vi "Autonomous Independent.vi"   [LabVIEW 2017]
doc: "This VI is called when autonomous begins, and will automatically be terminated when autonomous ends. You can carry out timed or sensor driven robot movement independently without needing to return to the caller."
uses:
  <vilib>/Rock Robotics/WPI/Utilities/WPI_GetSetVariantRefNum.vi
  <vilib>/Rock Robotics/Network Tables/NT Read String.vi
  Robot Global Data.vi
  <vilib>/Rock Robotics/Network Tables/NT Write Numeric Array.vi
  <vilib>/Rock Robotics/WPI/RobotDrive/WPI_RobotDriveMecanumDrive_Cartesian.vi
panel:
  # "Be sure to right-click and choose Data Operations>>Make Current Value default if you want to save the array values with the VI"
types:
  T1 = typedef "WPI_JoystickDevRef.ctl" = cluster{"Device":T2}
  T2 = typedef "WPI_JoystickDeviceEnum.ctl" = enum16{"USB 0", "USB 1", "USB 2", "USB 3", "USB 4", "USB 5"}
  T3 = typedef "WPI_RobotDriveDevRef.ctl" = cluster{"DevStatus":errorcluster, "Motors[]":T4[], "Square Inputs":bool, "Max Output":dbl}
  T4 = typedef "WPI_MotorControlDeviceRef.ctl" = cluster{"DeviceStatus":errorcluster, "Type":T5, "PWM":cluster{"PWM Channel":T6, "DeadBand":T7}, "CAN":cluster{"Device Number":u8, "SetOutput VI Ref":variant, "GetOutput VI Ref":variant, "Enable VI Ref":variant, "Disable VI Ref":variant, "Data":variant}, "Invert":bool, "DIO PWM":cluster{"PWM \"Enable\" Channel":T6, "DIOChannel":T8, "PWM Rate":dbl}}
  T5 = typedef "WPI_MotorControlType.ctl" = enum16{"PWM", "CAN", "DIO PWM"}
  T6 = typedef "FPGA_DIOPWMChannel.ctl" = enum8{"PWM 0", "PWM 1", "PWM 2", "PWM 3", "PWM 4", "PWM 5", "PWM 6", "PWM 7", "PWM 8", "PWM 9", "PWM MXP 0", "PWM MXP 1", "PWM MXP 2", "PWM MXP 3", "PWM MXP 4", "PWM MXP 5", "PWM MXP 6", "PWM MXP 7", "PWM MXP 8", "PWM MXP 9", "Invalid"}
  T7 = typedef "WPI_PWMDeadband.ctl" = cluster{"Name":string, "maxPositivePwm":i32, "minPositivePwm":i32, "centerPwm":i32, "maxNegativePwm":i32, "minNegativePwm":i32, "angularRange":u16}
  T8 = typedef "FPGA_DIOChannel.ctl" = enum8{"DIO 0", "DIO 1", "DIO 2", "DIO 3", "DIO 4", "DIO 5", "DIO 6", "DIO 7", "DIO 8", "DIO 9", "DIO MXP 0", "DIO MXP 1", "DIO MXP 2", "DIO MXP 3", "DIO MXP 4", "DIO MXP 5", "DIO MXP 6", "DIO MXP 7", "DIO MXP 8", "DIO MXP 9", "DIO MXP 10", "DIO MXP 11", "DIO MXP 12", "DIO MXP 13", "DIO MXP 14", "DIO MXP 15", "SPI Port CS1", "SPI Port CS2", "SPI Port CS3", "SPI Port MISO", "SPI Port MOSI", "Invalid"}
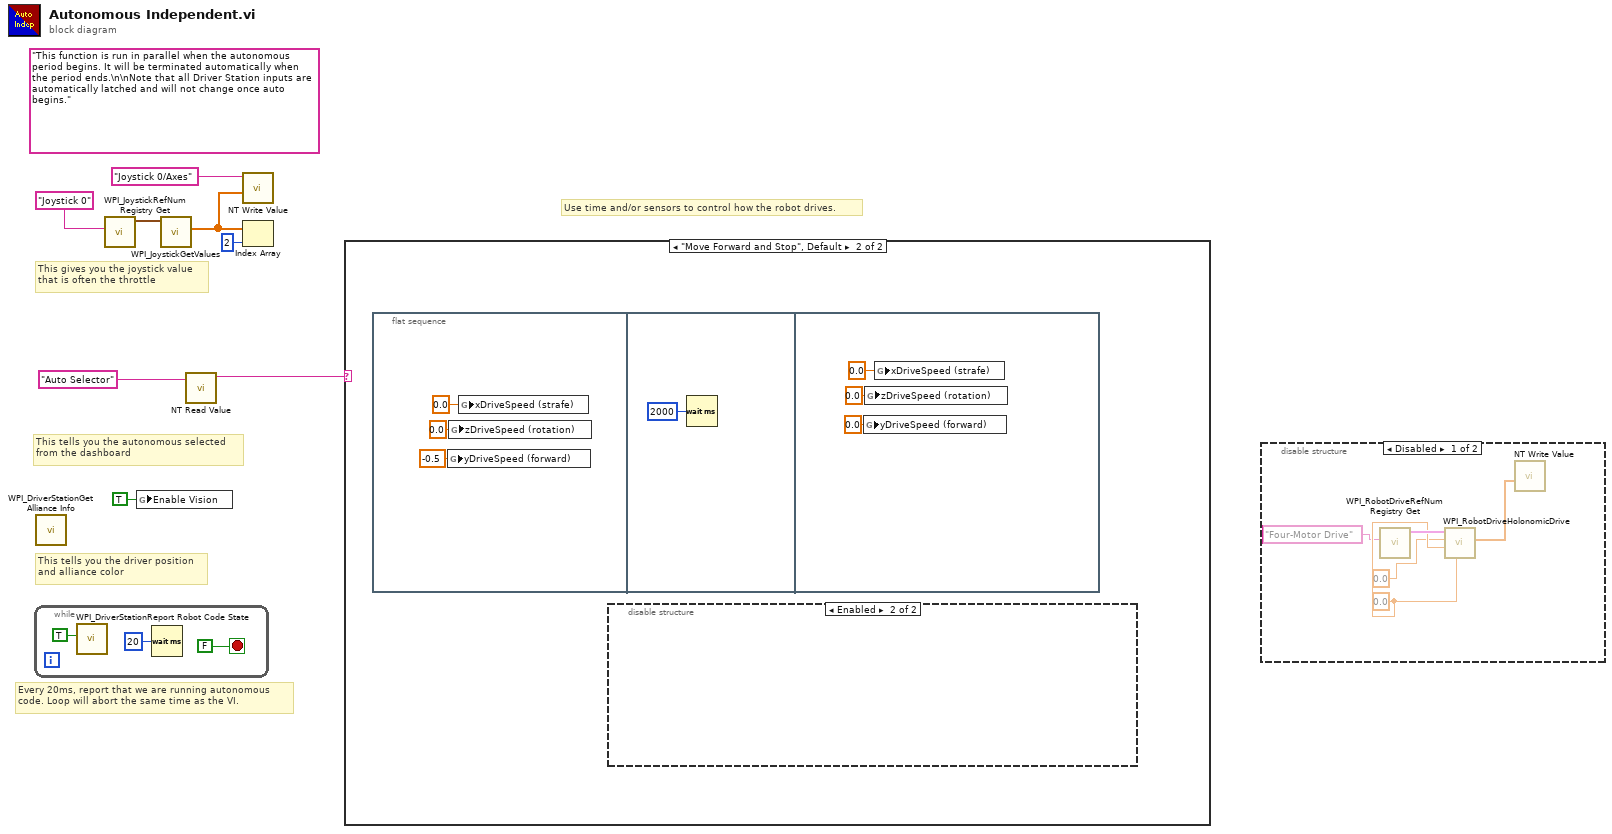
[diagram p0: block diagram]
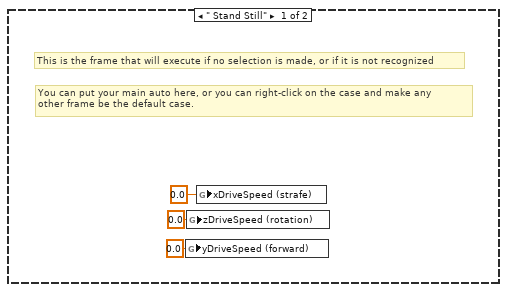
[diagram p3: hidden frame]
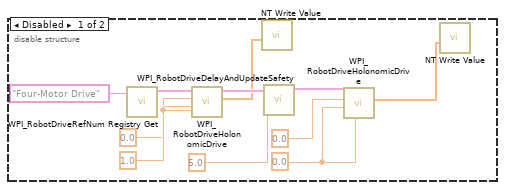
[diagram p4: hidden frame]
diagram:
  (unwired) "This function is run in parallel when the autonomous period begins. It will be terminated automatically when the period ends.\n\nNote that all Driver Station inputs are automatically latched and will not change once auto begins."
  # "This tells you the autonomous selected\nfrom the dashboard"
  # "Every 20ms, report that we are running autonomous\ncode. Loop will abort the same time as the VI."
  # "This gives you the joystick value\nthat is often the throttle"
  # "Use time and/or sensors to control how the robot drives."
  # "This tells you the driver position\nand alliance color"
  n1 = while {
    stop <- FALSE stop-if-true
    n2 = call <vilib>:"WPI_DriverStationReport Robot Code State.vi"("Autonomous"=TRUE) -> ()  [unwired: 10 in, 1 out]
    n3 = Wait (ms)(milliseconds to wait=u32 20) -> ()  [unwired: 1 out]
  }
  n4 = call <vilib>:"WPI_DriverStationGet Alliance Info.vi"() -> ()  [unwired: 12 out]
  n5 = call <vilib>:"WPI_JoystickRefNum Registry Get.vi"("refnum name"="Joystick 0") -> ("JoystickDevRef"=w7:T1)  [unwired: 1 in, 9 out]
  n6 = global write "Robot Global Data.vi" "Enable Vision"(TRUE ("Enable Vision")) -> ()
  n7 = call <vilib>:"WPI_JoystickGetValues.vi"("JoystickDevRef"=w7) -> ("Axes"=w3:dbl[])  [unwired: 6 in, 4 out]
  n8 = call-poly <vilib>:"NT Read Value.vi"("Name"="Auto Selector") -> ("String"=w4:string)  [unwired: 9 in, 1 out]
  n9 = call-poly <vilib>:"NT Write Value.vi"("Numeric Array"=w3, "Name"="Joystick 0/Axes") -> ()  [unwired: 9 in, 1 out]
  n10 = Index Array(array=w3, index=2) -> ()  [unwired: 1 out]
  n11 = case shown="\"Move Forward and Stop\", Default" w4 {
    frame " Stand Still" {
      # "You can put your main auto here, or you can right-click on the case and make any\nother frame be the default case."
      # "This is the frame that will execute if no selection is made, or if it is not recognized"
      n12 = global write "Robot Global Data.vi" "yDriveSpeed (forward)"(0.0 ("xDriveSpeed (strafe)")) -> ()
      n13 = global write "Robot Global Data.vi" "zDriveSpeed (rotation)"(0.0 ("xDriveSpeed (strafe)")) -> ()
      n14 = global write "Robot Global Data.vi" "xDriveSpeed (strafe)"(0.0 ("xDriveSpeed (strafe)")) -> ()
    }
    frame "Move Forward and Stop", Default {
      n15 = flat-sequence {
        frame #0 {
          n16 = global write "Robot Global Data.vi" "yDriveSpeed (forward)"(-0.5 ("xDriveSpeed (strafe)")) -> ()
          n17 = global write "Robot Global Data.vi" "zDriveSpeed (rotation)"(0.0 ("xDriveSpeed (strafe)")) -> ()
          n18 = global write "Robot Global Data.vi" "xDriveSpeed (strafe)"(0.0 ("xDriveSpeed (strafe)")) -> ()
        }
        frame #1 {
          n19 = Wait (ms)(milliseconds to wait=u32 2000) -> ()  [unwired: 1 out]
        }
        frame #2 {
          n20 = global write "Robot Global Data.vi" "yDriveSpeed (forward)"(0.0 ("xDriveSpeed (strafe)")) -> ()
          n21 = global write "Robot Global Data.vi" "zDriveSpeed (rotation)"(0.0 ("xDriveSpeed (strafe)")) -> ()
          n22 = global write "Robot Global Data.vi" "xDriveSpeed (strafe)"(0.0 ("xDriveSpeed (strafe)")) -> ()
        }
      }
      n23 = disable-structure shown="Enabled" {
        frame Disabled {
          w16 = 0.0 ("Y axis value")
          w15 = 0.0 ("X axis value")
          n24 = call <vilib>:"WPI_RobotDriveRefNum Registry Get.vi"("refnum name"="Four-Motor Drive") -> ("RobotDriveDevRef"=w24:T3)  [unwired: 9 in, 1 out]
          n25 = call-poly <vilib>:"WPI_RobotDriveHolonomicDrive.vi"("Rotation"=w15, "Y"=1.0 ("Y axis value"), "X"=w15, "RobotDriveDevRef"=w24) -> ("Motor Values"=w20:dbl[], "RobotDriveDevRef"=w22:T3)  [unwired: 5 in, 1 out]
          n26 = call-poly <vilib>:"NT Write Value.vi"("Numeric Array"=w20) -> ()  [unwired: 10 in, 1 out]
          n27 = call <vilib>:"WPI_RobotDriveDelayAndUpdateSafety.vi"("Delay (s)"=5.0, "RobotDriveDevRef"=w22) -> ("RobotDriveDevRef 2"=w19:T3)  [unwired: 8 in, 1 out]
          n28 = call-poly <vilib>:"WPI_RobotDriveHolonomicDrive.vi"("Rotation"=w16, "Y"=w16, "X"=0.0 ("X axis value"), "RobotDriveDevRef"=w19) -> ("Motor Values"=w17:dbl[])  [unwired: 5 in, 2 out]
          n29 = call-poly <vilib>:"NT Write Value.vi"("Numeric Array"=w17) -> ()  [unwired: 10 in, 1 out]
        }
        frame Enabled {
        }
      }
    }
  }
  n30 = disable-structure shown="Disabled" {
    frame Disabled {
      w35 = 0.0 ("Y axis value")
      n31 = call <vilib>:"WPI_RobotDriveRefNum Registry Get.vi"("refnum name"="Four-Motor Drive") -> ("RobotDriveDevRef"=w36:T3)  [unwired: 9 in, 1 out]
      n32 = call-poly <vilib>:"WPI_RobotDriveHolonomicDrive.vi"("Rotation"=w35, "Y"=w35, "X"=0.0 ("X axis value"), "RobotDriveDevRef"=w36) -> ("Motor Values"=w37:dbl[])  [unwired: 5 in, 2 out]
      n33 = call-poly <vilib>:"NT Write Value.vi"("Numeric Array"=w37) -> ()  [unwired: 10 in, 1 out]
    }
    frame Enabled {
    }
  }
